vi "Main - Copy.vi"() -> ()   [LabVIEW 2014]
uses:
  <vilib>/myRIO/Common/Instrument Driver Framework/myRIO v1.0/PWM/vis/myRIO v1.1 Open PWM.vi
  <vilib>/myRIO/Common/Instrument Driver Framework/myRIO v1.0/UART/vis/myRIO v1.0 Close UART.vi
  <vilib>/myRIO/Common/Instrument Driver Framework/Utilities/vis/Validate Channels.vi
  <vilib>/myRIO/Common/Instrument Driver Framework/myRIO v1.0/PWM/vis/myRIO v1.0 Reserve PWM.vi
  <vilib>/myRIO/Common/Instrument Driver Framework/myRIO v1.0/PWM/vis/myRIO v1.0 Build MUX Configuration PWM.vi
  <vilib>/myRIO/Common/Instrument Driver Framework/myRIO v1.0/Resource Manager/vis/myRIO v1.0 Reserve Channel List.vi
  <vilib>/myRIO/Common/Instrument Driver Framework/myRIO v1.0/Resource Manager/vis/myRIO v1.0 Create Configuration List.vi
  <vilib>/myRIO/Common/Instrument Driver Framework/myRIO v1.0/Resource Manager/vis/myRIO v1.0 Reserve Channel.vi
  <vilib>/myRIO/Common/Instrument Driver Framework/myRIO v1.0/Resource Manager/vis/myRIO v1.0 Unreserve Channel.vi
  <vilib>/myRIO/Common/Instrument Driver Framework/myRIO v1.0/Resource Manager/vis/myRIO v1.0 Build Mutex Name.vi
  <vilib>/Utility/VariantDataType/GetNumericInfo.vi
  <vilib>/Utility/error.llb/Error Cluster From Error Code.vi
  <vilib>/myRIO/Common/Instrument Driver Framework/myRIO v1.0/myRIO v1.1 Open.vi
  <vilib>/myRIO/Common/Instrument Driver Framework/Utilities/vis/IO Manager.vi
  <vilib>/myRIO/Common/Instrument Driver Framework/Utilities/vis/Configuration Manager.vi
  <vilib>/myRIO/Common/Instrument Driver Framework/myRIO v1.0/Resource Manager/vis/myRIO v1.0 Configure IO.vi
  <vilib>/myRIO/Common/Instrument Driver Framework/myRIO v1.0/myRIO v1.0 Close.vi
  <vilib>/myRIO/Common/Instrument Driver Framework/myRIO v1.0/PWM/vis/myRIO v1.0 Write PWM.vi
  <vilib>/myRIO/Common/Instrument Driver Framework/Utilities/vis/FPGA Ref Manager.vi
  <vilib>/myRIO/Common/Instrument Driver Framework/myRIO v1.0/myRIO v1.0 Reset FPGA.vi
  <vilib>/myRIO/Common/Instrument Driver Framework/myRIO v1.0/IRQ/vis/myRIO v1.0 IRQ Info FGV.vi
  <vilib>/myRIO/Common/Instrument Driver Framework/myRIO v1.0/IRQ/vis/myRIO v1.0 Timer IRQ Info FGV.vi
  <vilib>/myRIO/Common/Instrument Driver Framework/myRIO v1.0/IRQ/vis/myRIO v1.0 ISR Agent.vi
  <vilib>/myRIO/Instrument Drivers/Utilities/Utilities.lvlib
  <vilib>/myRIO/Instrument Drivers/Onboard IO/PWM/PWM.lvlib
panel:
  out "String":string
  in  "null offset":bool
  in  "freq [Hz]":dbl=50.0
  in  "position [%FS]":dbl(slide) scale=-200.0..200.0
  in  "PWM channel":tag="B/PWM0"
  out "error out":errorcluster
  in  "Stop Button":bool
  # "Overview: The myRIO Project template acquires acceleration data from the onboard accelerometer and displays the changes of acceleration values in a waveform chart.\nInstructions:\n1. Check the myRIO target IP Address in the project and make sure the target IP Address is correct. \n2. Run the VI."
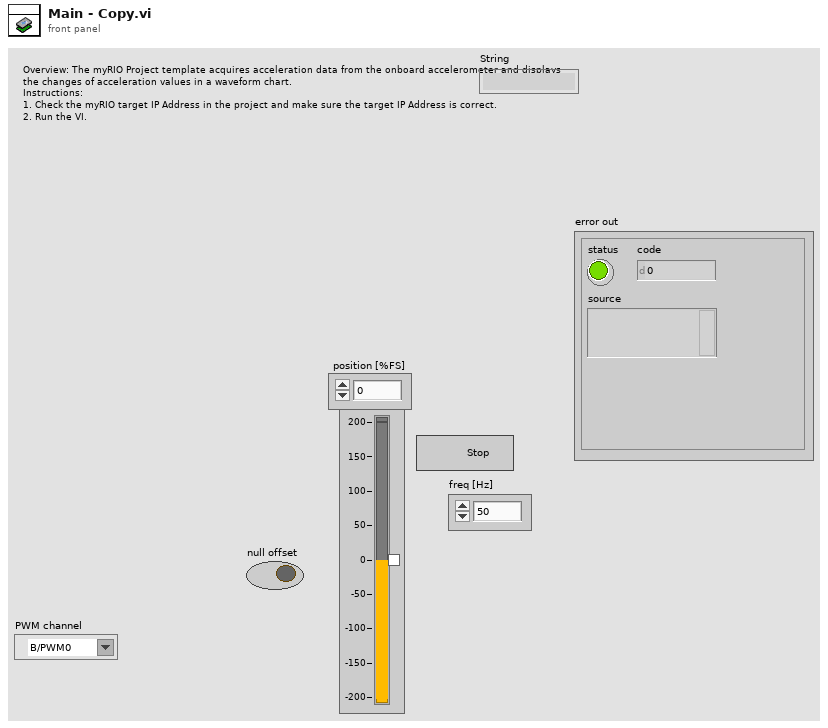
[diagram p1: front panel]
types:
  T1 = typedef "PWM.lvlib/PWM Reference.ctl" = cluster{"myRIO Reference":T2, "PWM Channels Enum":T6, "PWM Configuration":T7}
  T2 = typedef "myRIO Generic Hardware Reference.ctl" = cluster{"myRIO Model":T3, "myRIO Hardware Reference":T4}
  T3 = typedef "Hardware Version Enum.ctl" = enum16{"Unknown", "myRIO-1900", "myRIO-1950"}
  T4 = typedef "myRIO v1.0 Reference.ctl" = cluster{"Generic FPGA Reference":T5, "Allow multiple opens":bool}
  T5 = typedef "Generic FPGA Reference.ctl" = refnum<k20>
  T6 = typedef "PWM Channels Enum.ctl" = enum16{"Not Connected", "C/PWM0", "C/PWM1", "A/PWM0", "A/PWM1", "A/PWM2", "B/PWM0", "B/PWM1", "B/PWM2"}
  T7 = typedef "PWM.lvlib/PWM Configuration.ctl" = cluster{"Frequency":dbl, "Duty Cycle":dbl}
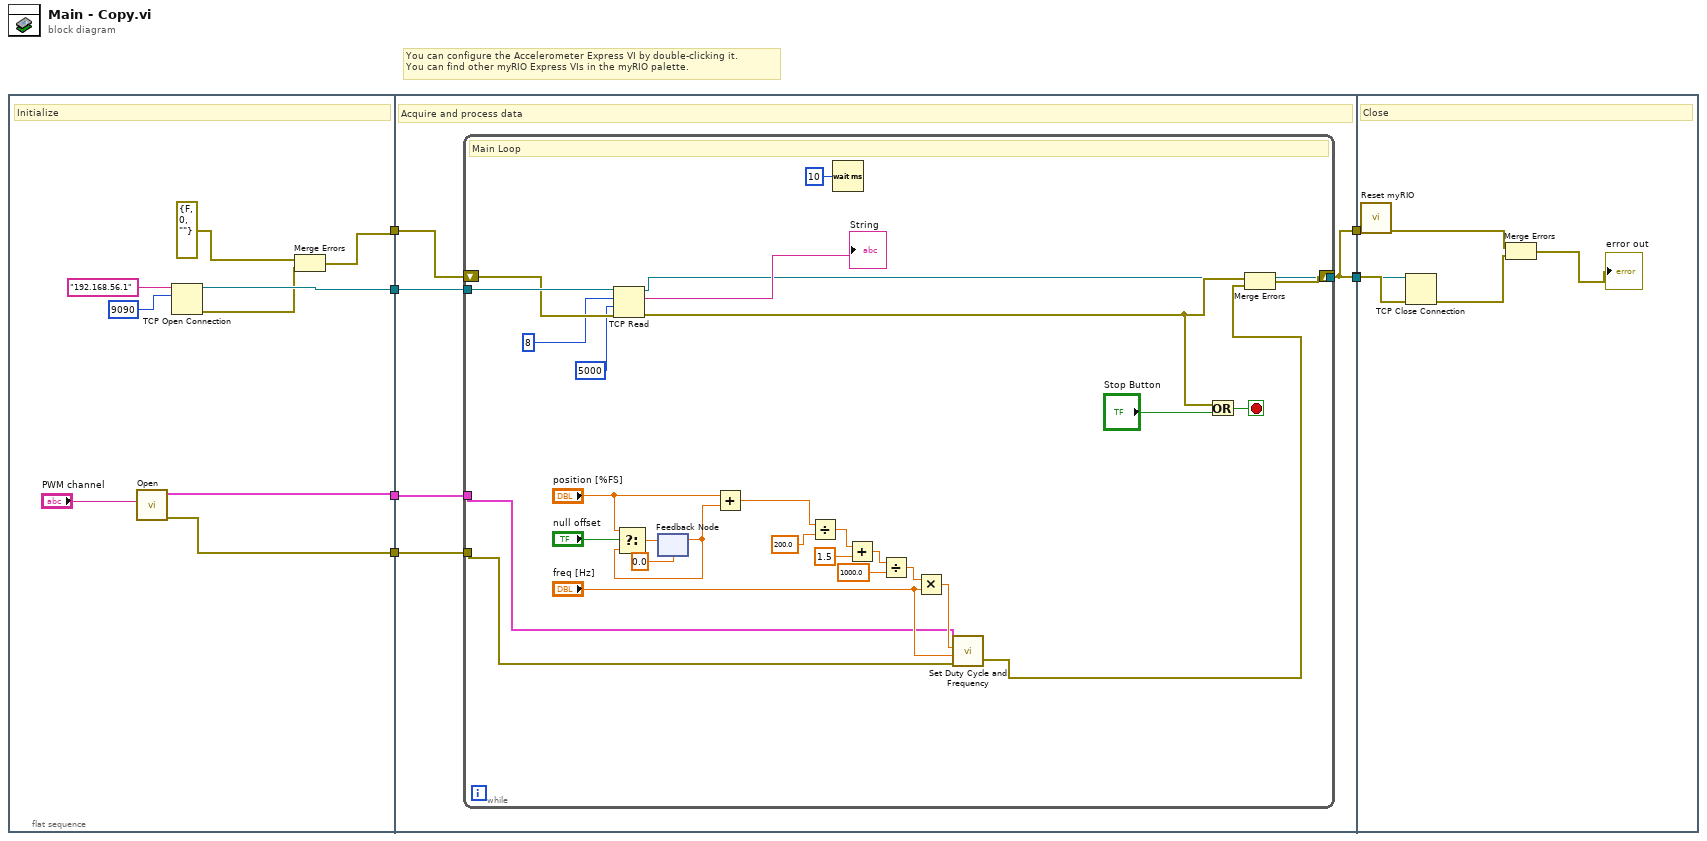
[diagram p0: block diagram]
diagram:
  # "You can configure the Accelerometer Express VI by double-clicking it.\nYou can find other myRIO Express VIs in the myRIO palette."
  n1 = flat-sequence {
    tunnel: [w8] -> w7
    tunnel: [w13] -> w5
    tunnel: [w12] -> w4
    tunnel: [w11] -> w3
    tunnel: w7 -> [w22]
    tunnel: [w18] -> w6
    tunnel: w5 -> [w21]
    tunnel: w4 -> [w20]
    tunnel: w3 -> [w19]
    tunnel: [w18] -> w2
    tunnel: [w17] -> w1
    tunnel: w6 -> [w56]
    tunnel: w2 -> [w55]
    tunnel: w1 -> [w54]
    frame #0 {
      # "Initialize"
      n2 = call <vilib>:"Open.vi"("Channel Name"="PWM channel") -> ("error out"=w13:errorcluster, "PWM Ref Out"=w12:T1)  [unwired: 9 in]
      n3 = TCP Open Connection(address="192.168.56.1", remote port or service name=u16 9090) -> (connection ID=w11:refnum<k5>, error out=w9:errorcluster)  [unwired: 3 in]
      n4 = Merge Errors(errorcluster {"status"=FALSE, "code"=0, "source"=""} ("error out"), w9) -> (w8:errorcluster)
    }
    frame #1 {
      # "Acquire and process data"
      n5 = while {
        shift-right: [w29] -> w18
        shift-left: w22 -> [w30]
        tunnel: w21 -> [w32]
        tunnel: w20 -> [w33]
        tunnel: w19 -> [w31]
        tunnel: [w23] -> w17
        stop <- w49 stop-if-true
        # "Main Loop"
        n6 = TCP Read(connection ID=w31, bytes to read=8, error in (no error)=w30, 9:5000) -> (connection ID out=w23:refnum<k5>, data out=→"String":string, error out=w27:errorcluster)  [unwired: 1 in]
        n7 = feedback #1(0.0 ("position [%FS]")) -> (w38:dbl)
        n8 = Select(t="position [%FS]", s="null offset", f=w38) -> (s? t:f=w40:dbl)
        n9 = feedback-in #1(w40) -> ()
        n10 = Add(x="position [%FS]", y=w38) -> (x+y=w39:dbl)
        n11 = Divide(x=w39, y=200.0) -> (x/y=w46:dbl)
        n12 = Wait (ms)(milliseconds to wait=u32 10) -> ()  [unwired: 1 out]
        n13 = Add(x=w46, y=1.5) -> (x+y=w44:dbl)
        n14 = Divide(x=w44, y=1000.0) -> (x/y=w36:dbl)
        n15 = Multiply(x=w36, y="freq [Hz]") -> (x*y=w34:dbl)
        n16 = call <vilib>:"Set Duty Cycle and Frequency.vi"("error in (no error)"=w32, "Frequency [Hz]"="freq [Hz]", "Duty Cycle"=w34, "PWM Ref In"=w33) -> ("error out"=w28:errorcluster)  [unwired: 5 in, 1 out]
        n17 = Or(x=w27, y="Stop Button") -> (x .or. y?=w49:bool)
        n18 = Merge Errors(w27, w28) -> (w29:errorcluster)
      }
    }
    frame #2 {
      # "Close"
      n19 = call <vilib>:"Reset myRIO.vi"("error in (no error)"=w56) -> ("error out"=w53:errorcluster)  [unwired: 10 in]
      n20 = TCP Close Connection(connection ID=w54, error in (no error)=w55) -> (error out=w52:errorcluster)  [unwired: 1 in, 1 out]
      n21 = Merge Errors(w53, w52) -> (→"error out":errorcluster)
    }
  }
